vi "BusUI.vi"() -> ()   [LabVIEW 2014, in "Bus.lvclass"]
doc: "UI that will be called when the node is selected."
uses:
  Bus.lvclass
  <vilib>/NI/Configuration Framework/Node/NodeRef.ctl
  <vilib>/NI/Configuration Framework/Node/NISE_CEF_Node.lvclass
  <vilib>/NI/AMC/Message Queue.ctl
  <vilib>/NI/AMC/Message.ctl
  <vilib>/NI/Tools/Keyed Array/KeyedArray.ctl
  <vilib>/NI/Configuration Framework/Node/UserEventRef.ctl
  <vilib>/NI/Configuration Framework/Controls/EventCluster.ctl
  Bus Configuration/SPI Configuration.ctl
  RIO Target/RIO Target.lvclass
  <vilib>/NI/Configuration Framework/Node/NISE_CEF_Node.lvclass/NISE_CEF_Node.ctl
  Bus.lvclass/Bus.ctl
  Bus Configuration/Bus Configuration.lvclass/Bus Configuration.ctl
  RIO Target Configuration/RIO Target Configuration.lvclass
  <vilib>/NI/AMC/Create Single Message.vi
  <vilib>/NI/AMC/Update Message Routing Info.vi
  <vilib>/NI/Configuration Framework/serializable configuration/read metadata property.vi
  <vilib>/NI/AMC/Send Message.vi
  <vilib>/NI/AMC/AMC.lvlib
  <vilib>/NI/Configuration Framework/serializable configuration/NISE_CEF_serializable configuration.lvclass
  Bus Configuration/Bus Configuration.lvclass
  <vilib>/NI/Tools/Keyed Array/Tools_KeyedArray.lvlib
  <vilib>/NI/Configuration Framework/NISE_CEF_TreeControl.lvlib
panel:
  in  "Replace Default DLU?":bool
  in  "Driver Logic Unit":path
  in  "Alias":string
  in  "SPI Configuration":T1
  in  "user event":T2
  in  "main queue":T3
  in  "node ref":T4
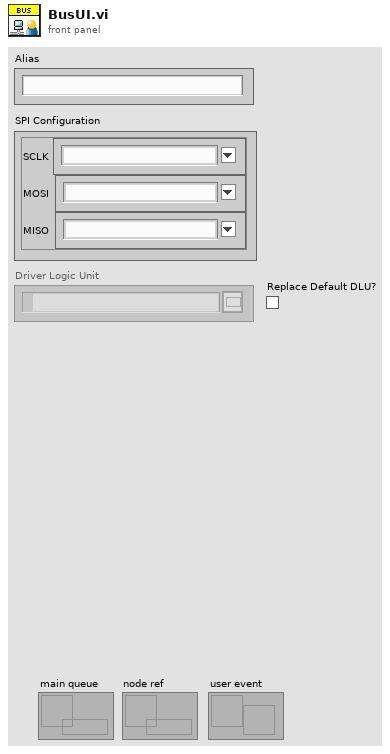
[diagram p1: front panel]
types:
  T1 = typedef "Bus Configuration.lvclass/SPI Configuration.ctl" = cluster{"SCLK":string, "MOSI":string, "MISO":string}
  T2 = typedef "NISE_CEF_Node.lvclass/UserEventRef.ctl" = refnum<user-event>
  T3 = typedef "AMC.lvlib/Message Queue.ctl" = refnum<queue>
  T4 = typedef "NISE_CEF_Node.lvclass/NodeRef.ctl" = refnum<data-value>
  T5 = enum8{"Enabled", "Disabled", "Disabled and Grayed Out"}
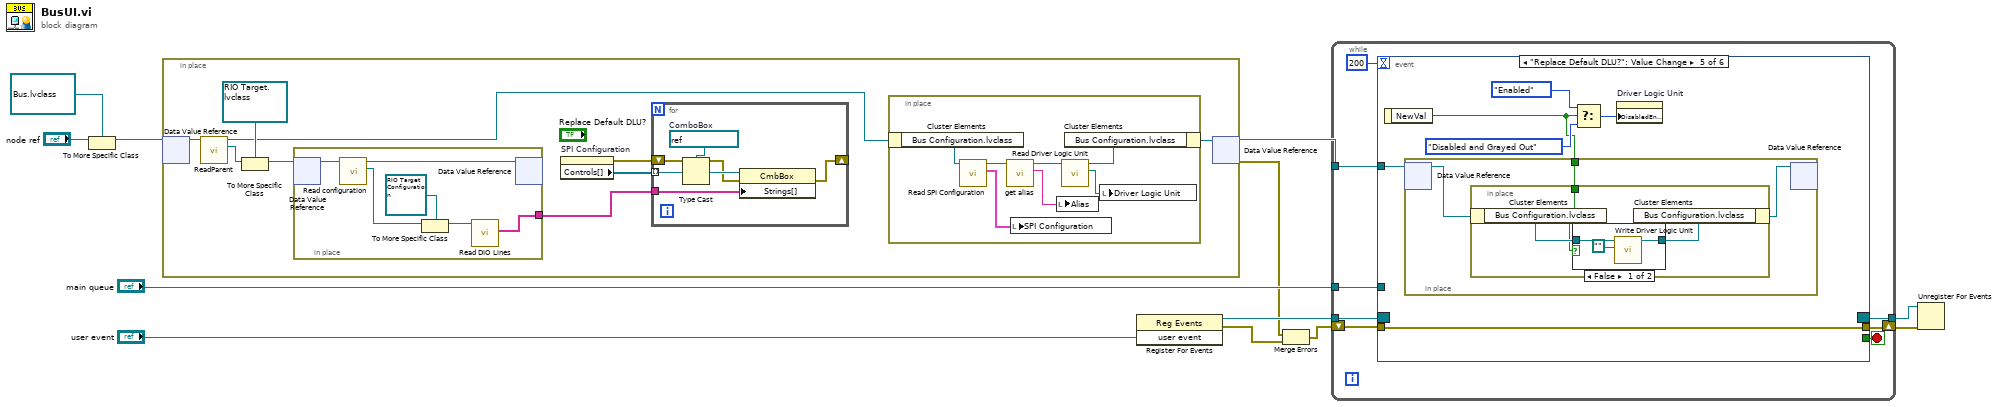
[diagram p0: block diagram]
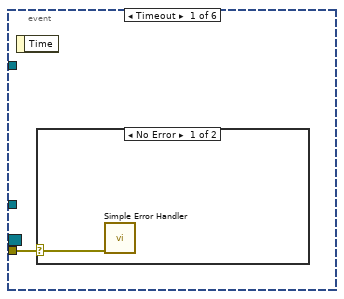
[diagram p2: hidden frame]
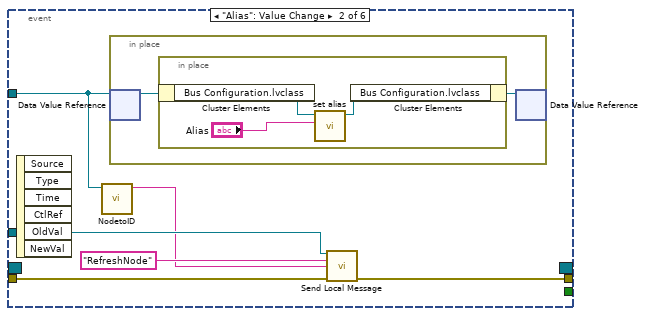
[diagram p4: hidden frame]
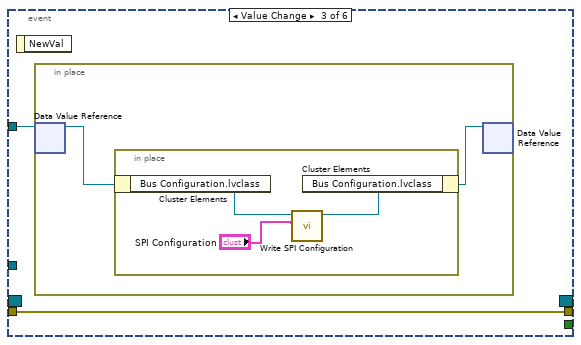
[diagram p5: hidden frame]
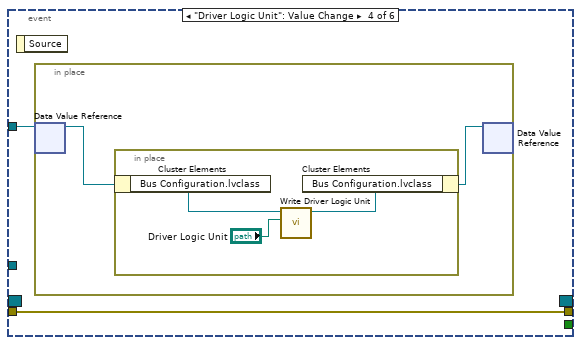
[diagram p6: hidden frame]
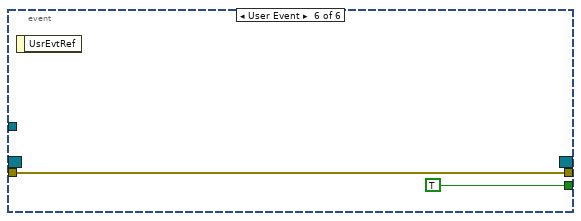
[diagram p8: hidden frame]
diagram:
  n1 = To More Specific Class(target class=refnum<data-value> refnum ("data value reference"), reference="node ref") -> (specific class reference=w2:refnum<data-value>)  [unwired: 1 in, 1 out]
  n2 = in-place {
    n3 = in-place-dvr #1(w2) -> (w21:refnum<class "Bus.lvclass">)  [unwired: 1 out]
    n4 = call <vilib>:"ReadParent.vi"("node in"=w21) -> ("parent"=w20:T4, "node out"=w15:refnum<class "Bus.lvclass">)  [unwired: 8 in, 1 out]
    n5 = To More Specific Class(target class=refnum<data-value> refnum ("data value reference"), reference=w20) -> (specific class reference=w18:refnum<data-value>)  [unwired: 1 in, 1 out]
    n6 = in-place {
      in-place-border: [w36] -> w13
      n7 = in-place-dvr #2(w18) -> (w40:refnum<class "RIO Target.lvclass">)  [unwired: 1 out]
      n8 = call-dynamic "Read configuration.vi"("RIO Target in"=w40) -> ("configuration"=w39:refnum<class "NISE_CEF_serializable configuration.lvclass">, "RIO Target out"=w35:refnum<class "RIO Target.lvclass">)  [unwired: 8 in, 1 out]
      n9 = To More Specific Class(target class=refnum<class "RIO Target Configuration.lvclass"> refnum ("RIO Target Configuration.lvclass"), reference=w39) -> (specific class reference=w37:refnum<class "RIO Target Configuration.lvclass">)  [unwired: 1 in, 1 out]
      n10 = call "Read DIO Lines.vi"("RIO Target Configuration in"=w37) -> ("DIO Lines"=w36:string[])  [unwired: 8 in, 2 out]
      n11 = in-place-dvr #2(w35) -> ()  [unwired: 2 out]
    }
    n12 = property on="SPI Configuration" class="Clust (strict)"() -> (error out=w17:errorcluster, "Controls[]"=w16:refnum<vi>[])  [unwired: 2 in, 1 out]
    n13 = for {
      tunnel: w16 -> [w34] mode=indexing
      shift-right: [w30] -> _
      shift-left: w17 -> [w31]
      tunnel: w13 -> [w29]
      w33 = refnum<vi> refnum  # ComboBox
      n14 = Type Cast(type=w33, x=w34) -> (*(type *) &x=w32:refnum<vi>)
      n15 = property class="CmbBox"(reference=w32, error in=w31, "Strings[]"=w29) -> (error out=w30:errorcluster)  [unwired: 1 out]
    }
    n16 = in-place {
      n17 = in-place-cluster #3(w15) -> ("Bus Configuration.lvclass"=w25:refnum<class "Bus Configuration.lvclass">)
      n18 = call "Read SPI Configuration.vi"("Bus Configuration in"=w25) -> ("SPI Configuration"=w28:T1, "Bus Configuration out"=w27:refnum<class "Bus Configuration.lvclass">)  [unwired: 8 in, 1 out]
      n19 = call <vilib>:"get alias.vi"("configuration in"=w27) -> ("alias"=w26:string, "configuration out"=w24:refnum<class "Bus Configuration.lvclass">)  [unwired: 8 in, 1 out]
      n20 = local write "SPI Configuration"(w28) -> ()
      n21 = local write "Alias"(w26) -> ()
      n22 = call "Read Driver Logic Unit.vi"("Bus Configuration in"=w24) -> ("Driver Logic Unit"=w22:path, "Bus Configuration out"=w23:refnum<class "Bus Configuration.lvclass">)  [unwired: 8 in, 1 out]
      n23 = in-place-cluster #3("Bus Configuration.lvclass"=w23) -> (w14:refnum<class "Bus.lvclass">)
      n24 = local write "Driver Logic Unit"(w22) -> ()
    }
    n25 = in-place-dvr #1(w14) -> (w12:refnum<data-value>, w6:errorcluster)
  }
  n26 = register-events("user event") -> (reference out=w9:refnum<event-registration>, error out=w5:errorcluster)  [unwired: 2 in]
  n27 = Merge Errors(w6, w5) -> (w4:errorcluster)
  n28 = while {
    tunnel: w12 -> [w48]
    tunnel: "main queue" -> [w47]
    tunnel: w9 -> [w45]
    tunnel: [w44] -> w8
    shift-right: [w42] -> w7
    shift-left: w4 -> [w41]
    stop <- w43 stop-if-true
    n29 = event shown="[4] \"Replace Default DLU?\": Value Change" {
      selector: w45 -> [_ _ _ _ _ _]
      dyn-events: [_ _ _ _ _ _] -> w44
      timeout: 200 -> [_ _ _ _ _ _]
      tunnel: w48 -> [_ w54 w62 w69 w80 _]
      tunnel: w47 -> [_ w55 _ _ _ _]
      tunnel: [_ _ _ _ _ TRUE] -> w43
      tunnel: [_ w52 w63 w70 w81 w92] -> w42
      tunnel: w41 -> [w49 w51 w63 w70 w81 w92]
      event Timeout {
        n30 = event-data() -> ()  [unwired: 1 in, 1 out]
        n31 = case shown="No Error" w49 {
          selector: w49 -> [w50 _]
          frame No Error {
            n32 = call <vilib>:"Simple Error Handler.vi"("error in (no error)"=w50) -> ()  [unwired: 4 in, 5 out]
          }
          frame Error {
          }
        }
      }
      event "Alias": Value Change {
        n33 = event-data() -> ()  [unwired: 1 in, 6 out]
        n34 = call <vilib>:"NodetoID.vi"("node ref"=w54) -> ("ID"=w53:string)  [unwired: 9 in, 1 out]
        n35 = in-place {
          n36 = in-place-dvr #4(w54) -> (w58:refnum<class "Bus.lvclass">)  [unwired: 1 out]
          n37 = in-place {
            n38 = in-place-cluster #5(w58) -> ("Bus Configuration.lvclass"=w61:refnum<class "Bus Configuration.lvclass">)
            n39 = call <vilib>:"set alias.vi"("alias"="Alias", "configuration in"=w61) -> ("configuration out"=w60:refnum<class "Bus Configuration.lvclass">)  [unwired: 8 in, 1 out]
            n40 = in-place-cluster #5("Bus Configuration.lvclass"=w60) -> (w57:refnum<class "Bus.lvclass">)
          }
          n41 = in-place-dvr #4(w57) -> ()  [unwired: 2 out]
        }
        n42 = call <vilib>:"Send Local Message.vi"("message queue in"=w55, "message name"="RefreshNode" ("Message Name"), "message value"=w53, "error in"=w51) -> ("error out"=w52:errorcluster)  [unwired: 9 in, 2 out]
      }
      event Value Change {
        n43 = event-data() -> ()  [unwired: 1 in, 1 out]
        n44 = in-place {
          n45 = in-place-dvr #6(w62) -> (w65:refnum<class "Bus.lvclass">)  [unwired: 1 out]
          n46 = in-place {
            n47 = in-place-cluster #7(w65) -> ("Bus Configuration.lvclass"=w67:refnum<class "Bus Configuration.lvclass">)
            n48 = call "Write SPI Configuration.vi"("SPI Configuration"="SPI Configuration", "Bus Configuration in"=w67) -> ("Bus Configuration out"=w66:refnum<class "Bus Configuration.lvclass">)  [unwired: 8 in, 1 out]
            n49 = in-place-cluster #7("Bus Configuration.lvclass"=w66) -> (w64:refnum<class "Bus.lvclass">)
          }
          n50 = in-place-dvr #6(w64) -> ()  [unwired: 2 out]
        }
      }
      event "Driver Logic Unit": Value Change {
        n51 = event-data() -> ()  [unwired: 1 in, 1 out]
        n52 = in-place {
          n53 = in-place-dvr #8(w69) -> (w72:refnum<class "Bus.lvclass">)  [unwired: 1 out]
          n54 = in-place {
            n55 = in-place-cluster #9(w72) -> ("Bus Configuration.lvclass"=w75:refnum<class "Bus Configuration.lvclass">)
            n56 = call "Write Driver Logic Unit.vi"("Driver Logic Unit"="Driver Logic Unit", "Bus Configuration in"=w75) -> ("Bus Configuration out"=w74:refnum<class "Bus Configuration.lvclass">)  [unwired: 8 in, 1 out]
            n57 = in-place-cluster #9("Bus Configuration.lvclass"=w74) -> (w71:refnum<class "Bus.lvclass">)
          }
          n58 = in-place-dvr #8(w71) -> ()  [unwired: 2 out]
        }
      }
      event "Replace Default DLU?": Value Change {
        n59 = event-data() -> ("NewVal"=w76:bool)  [unwired: 1 in]
        n60 = in-place {
          in-place-border: w76 -> [w82]
          n61 = in-place-dvr #10(w80) -> (w84:refnum<class "Bus.lvclass">)  [unwired: 1 out]
          n62 = in-place {
            in-place-border: w82 -> [w85]
            n63 = in-place-cluster #11(w84) -> ("Bus Configuration.lvclass"=w87:refnum<class "Bus Configuration.lvclass">)
            n64 = case shown="False" w85 {
              tunnel: w87 -> [w90 w91]
              tunnel: [w89 w91] -> w86
              frame False {
                n65 = call "Write Driver Logic Unit.vi"("Driver Logic Unit"=path "", "Bus Configuration in"=w90) -> ("Bus Configuration out"=w89:refnum<class "Bus Configuration.lvclass">)  [unwired: 8 in, 1 out]
              }
              frame True {
              }
            }
            n66 = in-place-cluster #11("Bus Configuration.lvclass"=w86) -> (w83:refnum<class "Bus.lvclass">)
          }
          n67 = in-place-dvr #10(w83) -> ()  [unwired: 2 out]
        }
        n68 = Select(t=T5."Enabled" ("Disabled"), s=w76, f=T5."Disabled and Grayed Out" ("Disabled")) -> (s? t:f=w77:T5)
        n69 = property on="Driver Logic Unit" class="Path"("DisabledEnum"=w77) -> ()  [unwired: 2 in, 2 out]
      }
      event User Event {
        n70 = event-data() -> ()  [unwired: 1 in, 1 out]
      }
    }
  }
  n71 = Unregister For Events(event registration refnum=w8, error in=w7) -> ()  [unwired: 1 out]
